vi "Write Recurrence Interval (s).vi"(8 "error in (no error)":errorcluster, 10 "Recurrence Interval (s)":u32, 11 "AExpense in":refnum<class "AExpense.lvclass">) -> (0 "error out":errorcluster, 3 "AExpense out":refnum<class "AExpense.lvclass">)   [LabVIEW 2020, in "AExpense.lvclass"]
uses:
  AExpense.lvclass
  AExpense.lvclass/AExpense.ctl
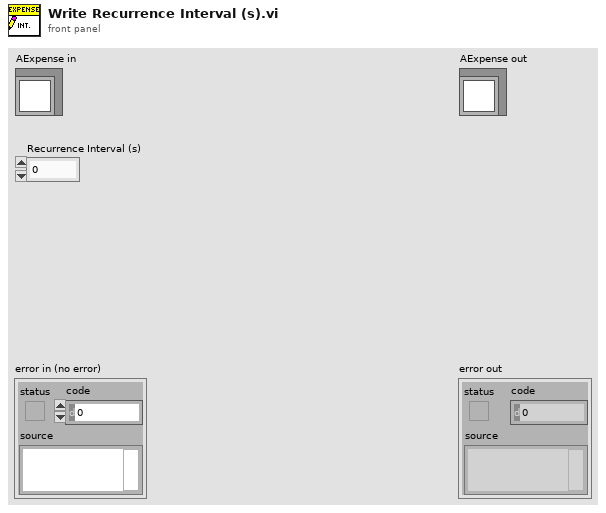
[diagram p1: front panel]
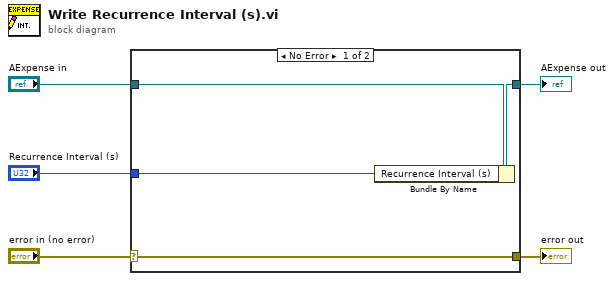
[diagram p0: block diagram]
diagram:
  n1 = case shown="No Error" "error in (no error)" {
    selector: "error in (no error)" -> [w9 w10]
    tunnel: [w9 w10] -> w4
    tunnel: [w7 w11] -> w2
    tunnel: "AExpense in" -> [w8 w11]
    tunnel: "Recurrence Interval (s)" -> [w6 _]
    frame No Error {
      n2 = Bundle By Name(cluster=w8, "Recurrence Interval (s)"=w6) -> (w7:refnum<class "AExpense.lvclass">)
    }
    frame Error {
    }
  }
  "error out" <- w4
  "AExpense out" <- w2
